vi "AddNewArmpressureReading.vi"() -> (2 "Cancel?":bool, 3 "output cluster":T1)   [LabVIEW 2013, in "main.lvlib"]
uses:
  main.lvlib
panel:
  out "AddArmPressure_TitleString":string="Tilføj armtryk"
  in  "Side":string(combo)="Left"
  in  "ArmPressureDia":dbl caption="Dia"
  in  "CancelReadingsBtn":bool
  in  "AddReadingsBtn":bool
  in  "ArmPuls":dbl caption="Puls"
  in  "ArmPressureSys":dbl caption="Sys"
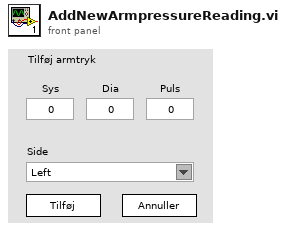
[diagram p1: front panel]
types:
  T1 = cluster{"ArmPressureSys":dbl, "ArmPressureDia":dbl, "ArmPuls":dbl, "Side":string}
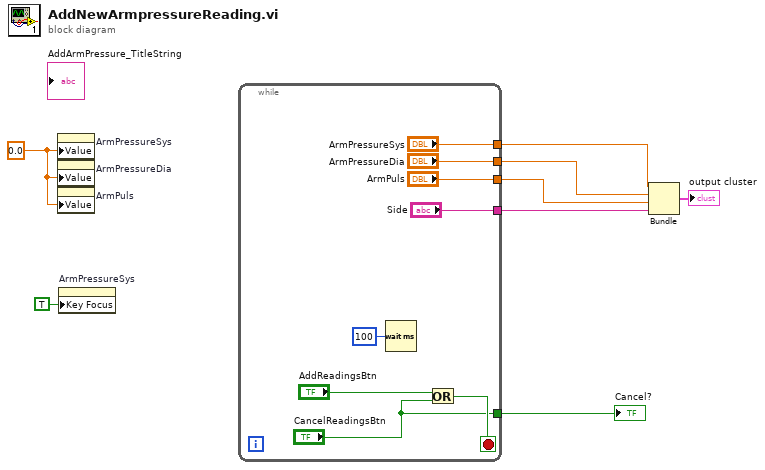
[diagram p0: block diagram]
diagram:
  w2 = 0.0 ("ArmPressureSys")
  n1 = property on="ArmPressureSys" class="DigNum (strict)"("Value"=w2) -> ()  [unwired: 2 in, 2 out]
  n2 = property on="ArmPressureDia" class="DigNum (strict)"("Value"=w2) -> ()  [unwired: 2 in, 2 out]
  n3 = property on="ArmPuls" class="DigNum (strict)"("Value"=w2) -> ()  [unwired: 2 in, 2 out]
  n4 = property on="ArmPressureSys" class="DigNum (strict)"("Key Focus"=TRUE) -> ()  [unwired: 2 in, 2 out]
  n5 = while {
    tunnel: ["CancelReadingsBtn"] -> w8
    tunnel: ["Side"] -> w4
    tunnel: ["ArmPressureSys"] -> w7
    tunnel: ["ArmPressureDia"] -> w6
    tunnel: ["ArmPuls"] -> w5
    stop <- w15 stop-if-true
    n6 = Wait (ms)(milliseconds to wait=u32 100) -> ()  [unwired: 1 out]
    n7 = Or(x="AddReadingsBtn", y="CancelReadingsBtn") -> (x .or. y?=w15:bool)
  }
  "Cancel?" <- w8
  n8 = Bundle("ArmPressureSys"=w7, "ArmPressureDia"=w6, "ArmPuls"=w5, "Side"=w4) -> (→"output cluster":T1)  [unwired: 1 in]
